vi "Set Speed.vi"(8 "error in (no error)":errorcluster, 10 "speed":dbl, 11 "VICI Settings In":T1 {"Pump Number" min=0.0 max=20.0 step=1.0}) -> (0 "error out":errorcluster, 1 "Connection Error":bool, 3 "VICI Settings Out":T1 {"Pump Number" min=0.0 max=20.0 step=1.0})   [LabVIEW 2018, in "VICI M50.lvlib"]
uses:
  VICI M50.lvlib
  Settings Cluster.ctl
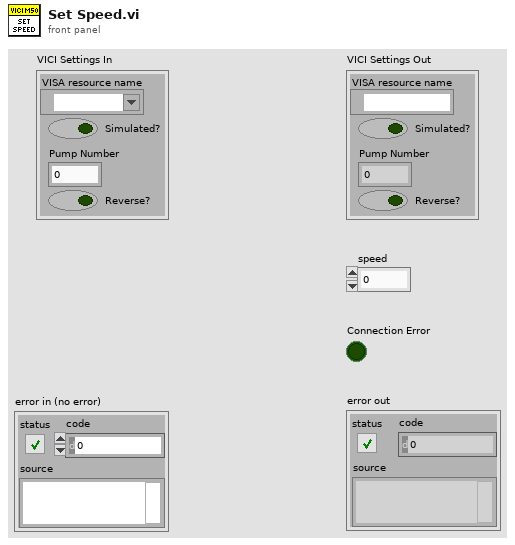
[diagram p1: front panel]
types:
  T1 = typedef "VICI M50.lvlib/Settings Cluster.ctl" = cluster{"VISA resource name":refnum<visa-resource-name>, "Simulated?":bool, "Pump Number":dbl, "Reverse?":bool}
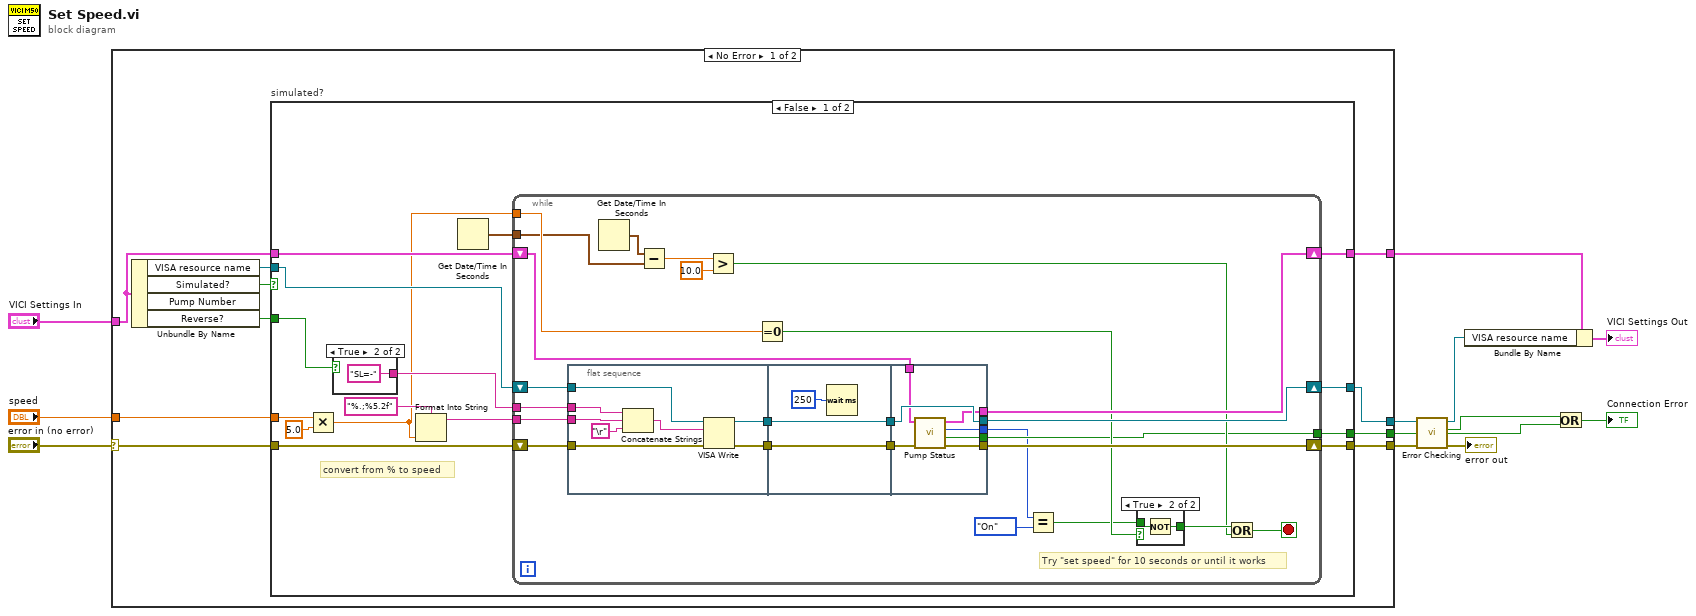
[diagram p0: block diagram]
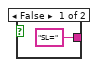
[diagram p3: hidden frame]
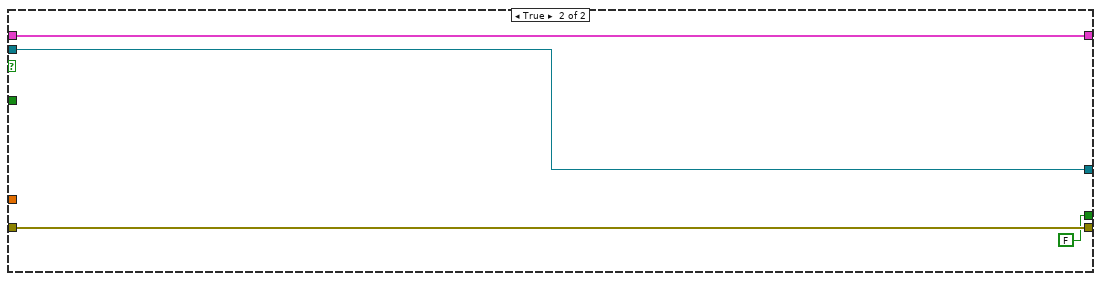
[diagram p4: hidden frame]
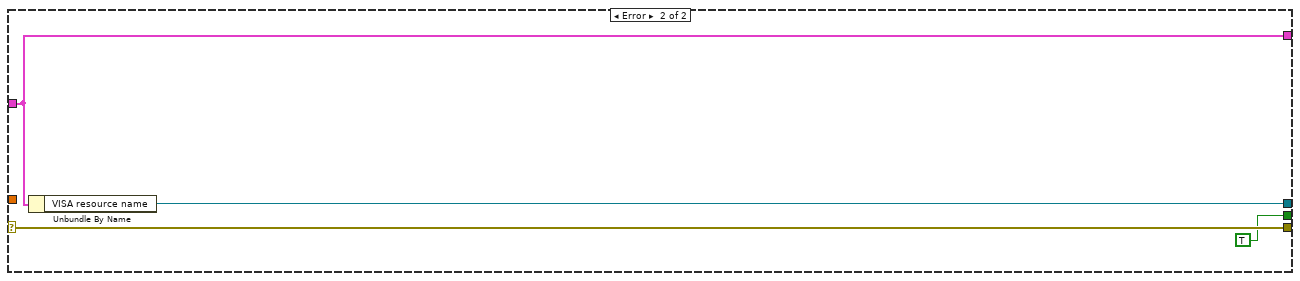
[diagram p5: hidden frame]
diagram:
  n1 = case shown="No Error" "error in (no error)" {
    selector: "error in (no error)" -> [w19 w93]
    tunnel: [w14 w92] -> w5
    tunnel: "VICI Settings In" -> [w15 w92]
    tunnel: "speed" -> [w18 _]
    tunnel: [w17 w91] -> w9
    tunnel: [w16 w93] -> w8
    tunnel: [w13 TRUE ("Connection Error")] -> w3
    frame No Error {
      n2 = Unbundle By Name(w15) -> ("VISA resource name"=w21:refnum<visa-resource-name>, "Simulated?"=w20:bool, "Reverse?"=w22:bool)  [unwired: 1 out]
      n3 = case "simulated?" shown="False" w20 {
        tunnel: [w35 w89] -> w17
        tunnel: w21 -> [w37 w89]
        tunnel: w19 -> [w36 w88]
        tunnel: [w34 w88] -> w16
        tunnel: w22 -> [w33 _]
        tunnel: w18 -> [w31 _]
        tunnel: w15 -> [w27 w87]
        tunnel: [w26 w87] -> w14
        tunnel: [w23 FALSE ("Connection Error")] -> w13
        frame False {
          # "convert from % to speed"
          n4 = Multiply(x=w31, y=5.0) -> (x*y=w25:dbl)
          n5 = case shown="True" w33 {
            tunnel: ["SL=" ("string") "SL=-" ("string")] -> w30
            frame False {
            }
            frame True {
            }
          }
          n6 = Format Into String(format string="%.;%5.2f", w25) -> (resulting string=w29:string)  [unwired: 2 in, 1 out]
          n7 = Get Date/Time In Seconds() -> (seconds since 1Jan1904=w24:timestamp)
          n8 = while {
            tunnel: w30 -> [w55]
            tunnel: w29 -> [w54]
            shift-right: [w57] -> w35
            shift-left: w37 -> [w42]
            shift-right: [w56] -> w34
            shift-left: w36 -> [w58]
            shift-right: [w52] -> w26
            shift-left: w27 -> [w53]
            tunnel: w25 -> [w51]
            tunnel: w24 -> [w44]
            tunnel: [w41] -> w23
            stop <- w47 stop-if-true
            # "Try \"set speed\" for 10 seconds or until it works"
            n9 = flat-sequence {
              tunnel: w42 -> [w73]
              tunnel: w58 -> [w72]
              tunnel: w55 -> [w69]
              tunnel: w54 -> [w68]
              tunnel: [w71] -> w62
              tunnel: [w70] -> w61
              tunnel: w62 -> [w76]
              tunnel: w61 -> [w75]
              tunnel: [w76] -> w60
              tunnel: [w75] -> w59
              tunnel: [w81] -> w56
              tunnel: [w83] -> w57
              tunnel: w60 -> [w83]
              tunnel: w59 -> [w82]
              tunnel: w53 -> [w80]
              tunnel: [w79] -> w52
              tunnel: [w78] -> w40
              tunnel: [w77] -> w41
              frame #0 {
                n10 = Concatenate Strings(w69, w68, "\r") -> (w67:string)
                n11 = VISA Write(VISA resource name=w73, write buffer=w67, error in (no error)=w72) -> (VISA resource name out=w71:refnum<visa-resource-name>, error out=w70:errorcluster)  [unwired: 1 out]
              }
              frame #1 {
                n12 = Wait (ms)(milliseconds to wait=u32 250) -> ()  [unwired: 1 out]
              }
              frame #2 {
                n13 = call "Pump Status.vi"("error in (no error)"=w82, "VICI Settings In"=w80) -> ("error out"=w81:errorcluster, "Connection Error"=w77:bool, "Pump On?"=w78:enum16{"Off", "On", "Not Initialized"}, "VICI Settings Out"=w79:T1)  [unwired: 6 in]
              }
            }
            n14 = Get Date/Time In Seconds() -> (seconds since 1Jan1904=w43:timestamp)
            n15 = Subtract(x=w43, y=w44) -> (x-y=w49:dbl)
            n16 = Greater?(x=w49, y=10.0) -> (0:w45:bool)
            n17 = Equal To 0?(x=w51) -> (x = 0?=w50:bool)
            n18 = Equal?(x=w40, y=enum16{"Off", "On", "Not Initialized"}."On") -> (x = y?=w39:bool)
            n19 = case shown="True" w50 {
              tunnel: [w63 w65] -> w48
              tunnel: w39 -> [w63 w64]
              frame False {
              }
              frame True {
                n20 = Not(x=w64) -> (.not. x?=w65:bool)
              }
            }
            n21 = Or(x=w48, y=w45) -> (x .or. y?=w47:bool)
          }
        }
        frame True {
        }
      }
    }
    frame Error {
      n22 = Unbundle By Name(w92) -> ("VISA resource name"=w91:refnum<visa-resource-name>)
    }
  }
  n23 = call "Error Checking.vi"("error in (no error)"=w8, "VISA resource name"=w9) -> ("error out"=→"error out":errorcluster, "Connection Error"=w2:bool, "VISA resource name"=w6:refnum<visa-resource-name>)  [unwired: 7 in]
  n24 = Bundle By Name(cluster=w5, "VISA resource name"=w6) -> (→"VICI Settings Out":T1)
  n25 = Or(x=w2, y=w3) -> (x .or. y?=→"Connection Error":bool)
